vi "Close Handle.vi"(8 "error in (no error)":errorcluster, 11 "HTTP Client reqwest in":refnum<class "HTTP Client reqwest.lvclass">) -> (0 "error out":errorcluster, 3 "HTTP Client reqwest out":refnum<class "HTTP Client reqwest.lvclass">)   [LabVIEW 2021, in "HTTP Client reqwest.lvclass"]
uses:
  HTTP Client reqwest.lvclass
  HTTP Client reqwest.lvclass/HTTP Client reqwest.ctl
  external/reqwest-rs-labview/lv_src/Client/Client.lvclass
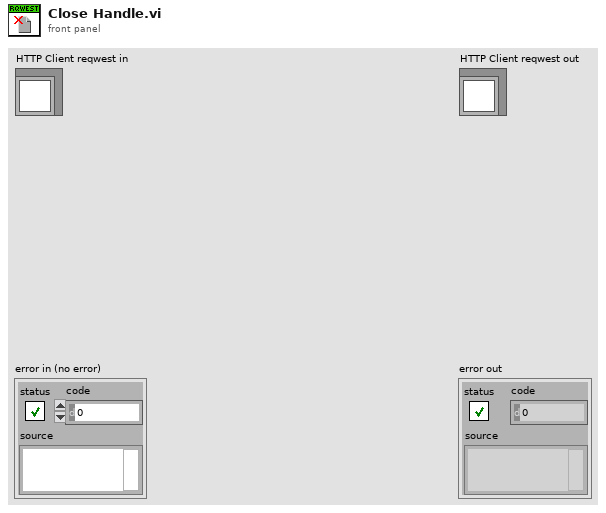
[diagram p1: front panel]
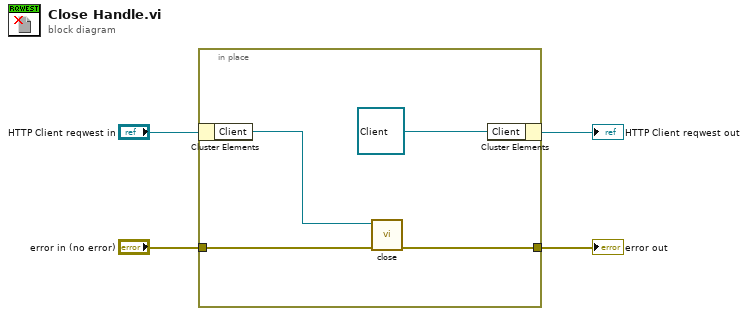
[diagram p0: block diagram]
diagram:
  n1 = in-place {
    in-place-border: "error in (no error)" -> [w8]
    in-place-border: [w7] -> w2
    n2 = in-place-cluster #1("HTTP Client reqwest in") -> ("Client"=w6:refnum<class "Client.lvclass">)
    n3 = call "close.vi"("error in (no error)"=w8, "Client in"=w6) -> ("error out"=w7:errorcluster)  [unwired: 9 in]
    n4 = in-place-cluster #1("Client"=refnum<class "Client.lvclass"> refnum) -> (→"HTTP Client reqwest out":refnum<class "HTTP Client reqwest.lvclass">)
  }
  "error out" <- w2
